vi "Make DLL Param(Read Batch Profile Req).vi"(1 "Read Batch Profile Req":T1 {"Batch Pos" items=["CURRENT"=0, "SPECIFY"=2, "COMMITED"=3, "NEWEST PROFILE"=4]}) -> (0 "pReq":T3 {"Batch Pos" items=["CURRENT"=0, "SPECIFY"=2, "COMMITED"=3, "NEWEST PROFILE"=4]})   [LabVIEW 2020, in "KEYENCE LJ-X8000A.lvlib"]
uses:
  KEYENCE LJ-X8000A.lvlib
  Public/Constants/Batch Pos.ctl
  Public/Clusters/Read Batch Profile Req.ctl
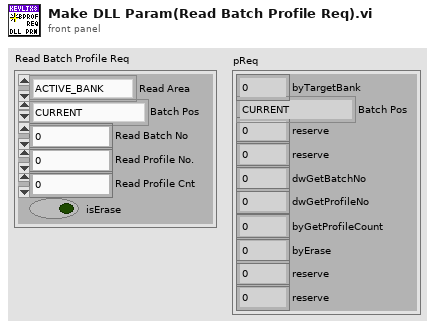
[diagram p1: front panel]
types:
  T1 = typedef "KEYENCE LJ-X8000A.lvlib/Read Batch Profile Req.ctl" = cluster{"Read Area":enum8{"ACTIVE_BANK", "INACTIVE_BANK"}, "Batch Pos":T2, "Read Batch No":u32, "Read Profile No.":u32, "Read Profile Cnt":u8, "isErase":bool}
  T2 = typedef "KEYENCE LJ-X8000A.lvlib/Batch Pos.ctl" = u8
  T3 = cluster{"byTargetBank":u8, "Batch Pos":T2, "reserve":u8, "reserve":u8, "dwGetBatchNo":u32, "dwGetProfileNo":u32, "byGetProfileCount":u8, "byErase":u8, "reserve":u8, "reserve":u8}
  T4 = cluster{"Read Area":enum8{"ACTIVE_BANK", "INACTIVE_BANK"}, "Batch Pos":T2, "reserve":u8, "reserve":u8, "Read Batch No":u32, "Read Profile No.":u32, "Read Profile Cnt":u8, u8, "reserve":u8, "reserve":u8}
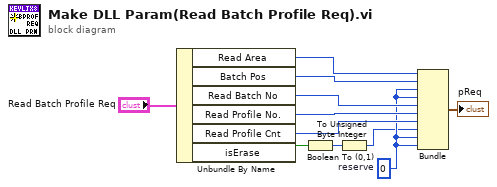
[diagram p0: block diagram]
diagram:
  w6 = u8 0  # reserve
  n1 = Unbundle By Name("Read Batch Profile Req") -> ("Read Area"=w1:enum8{"ACTIVE_BANK", "INACTIVE_BANK"}, "Batch Pos"=w11:T2, "Read Batch No"=w10:u32, "Read Profile No."=w9:u32, "Read Profile Cnt"=w7:u8, "isErase"=w5:bool)
  n2 = Boolean To (0,1)(Boolean=w5) -> (0, 1=w8:i16)
  n3 = To Unsigned Byte Integer(number=w8) -> (unsigned 8bit integer=w4:u8)
  n4 = Bundle("Read Area"=w1, "Batch Pos"=w11, "reserve"=w6, "reserve"=w6, "Read Batch No"=w10, "Read Profile No."=w9, "Read Profile Cnt"=w7, w4, "reserve"=w6, "reserve"=w6) -> (→"pReq":T4)  [unwired: 1 in]
